vi "Dequeue Message (poly).vi"   [LabVIEW 2018]
uses:
  Message Queue.lvlib
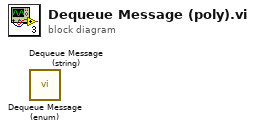
[diagram p0: block diagram]
diagram:
  n1 = call "Dequeue Message (enum).vi"() -> ()  [unwired: 9 in, 3 out]
  n2 = call "Dequeue Message (string).vi"() -> ()  [unwired: 8 in, 4 out]
